vi "CIMAQ_imagesize_seteven.vi"(11 "Refnum in":T1) -> (1 "Numeric":i32, 2 "Numeric 2":i32, 3 "Refnum out":T1)   [LabVIEW 2014]
uses:
  <vilib>/vision/Image Controls.llb/IMAQ Image.ctl
  <vilib>/vision/NI_Vision_Development_Module.lvlib
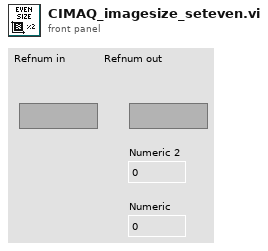
[diagram p1: front panel]
types:
  T1 = typedef "IMAQ Image.ctl" = refnum<image>
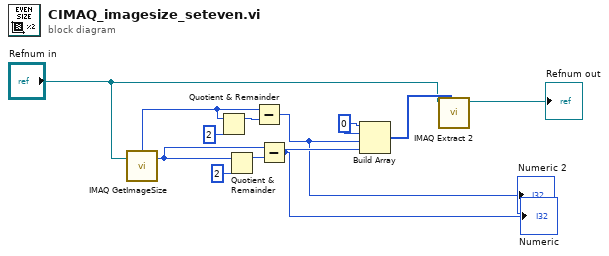
[diagram p0: block diagram]
diagram:
  w8 = 0 ("y")
  n1 = call "IMAQ GetImageSize"("Image"="Refnum in") -> ("Y Resolution"=w2:i32, "X Resolution"=w7:i32)  [unwired: 3 in, 1 out]
  n2 = Quotient & Remainder(x=w7, y=2) -> (x-y*floor(x/y)=w4:i32)  [unwired: 1 out]
  n3 = Quotient & Remainder(x=w2, y=2) -> (x-y*floor(x/y)=w3:i32)  [unwired: 1 out]
  n4 = Subtract(x=w7, y=w4) -> (x-y=w11:i32)
  "Numeric 2" <- w11
  n5 = Subtract(x=w2, y=w3) -> (x-y=w12:i32)
  "Numeric" <- w12
  n6 = Build Array(w8, w8, w11, w12) -> (w9:i32[])
  n7 = call "IMAQ Extract 2"("Optional Rectangle"=w9, "Image Src"="Refnum in") -> ("Image Dst Out"=→"Refnum out":T1)  [unwired: 8 in, 1 out]
